vi "Shared Variables CD 2.0 Initialization VI.vi"(8 "error in (no error)":errorcluster, 10 "Custom XML":string, 11 "Device Item Ref in":T1 format="%.0x") -> (0 "error out":errorcluster, 3 "Device Item Ref out":T1 format="%.0x")   [LabVIEW 2017, in "Shared Variables CD 2.0 Configuration.lvlib"]
uses:
  Shared Variables CD 2.0 Configuration.lvlib
  <vilib>/NI Veristand/Custom Device API/Custom Device Item Ref.ctl
  <vilib>/NI Veristand/Custom Device API/Custom Device Channel.ctl
  <vilib>/NI Veristand/Custom Device API/Custom Device Channel Type.ctl
  Shared/Shared Variables CD 2.0 GUID Lookup.vi
  Shared/SV Global.vi
  <vilib>/NI VeriStand/Custom Device API/Custom Device API.lvlib
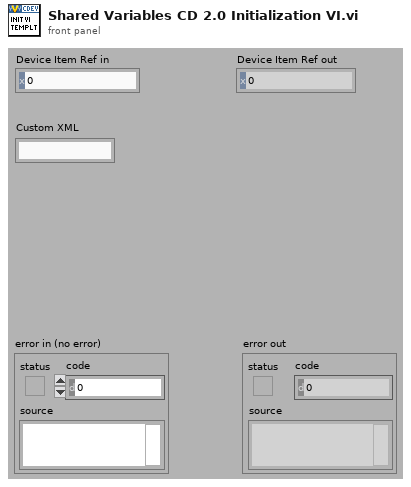
[diagram p1: front panel]
types:
  T1 = typedef "Custom Device API.lvlib/Custom Device Item Ref.ctl" = u64
  T2 = typedef "Custom Device API.lvlib/Custom Device Channel.ctl" = cluster{"Type":T3, "Units":string, "Default Value":dbl, "Faultable":bool, "Scalable":bool}
  T3 = typedef "Custom Device API.lvlib/Custom Device Channel Type.ctl" = enum16{"Input", "Output"}
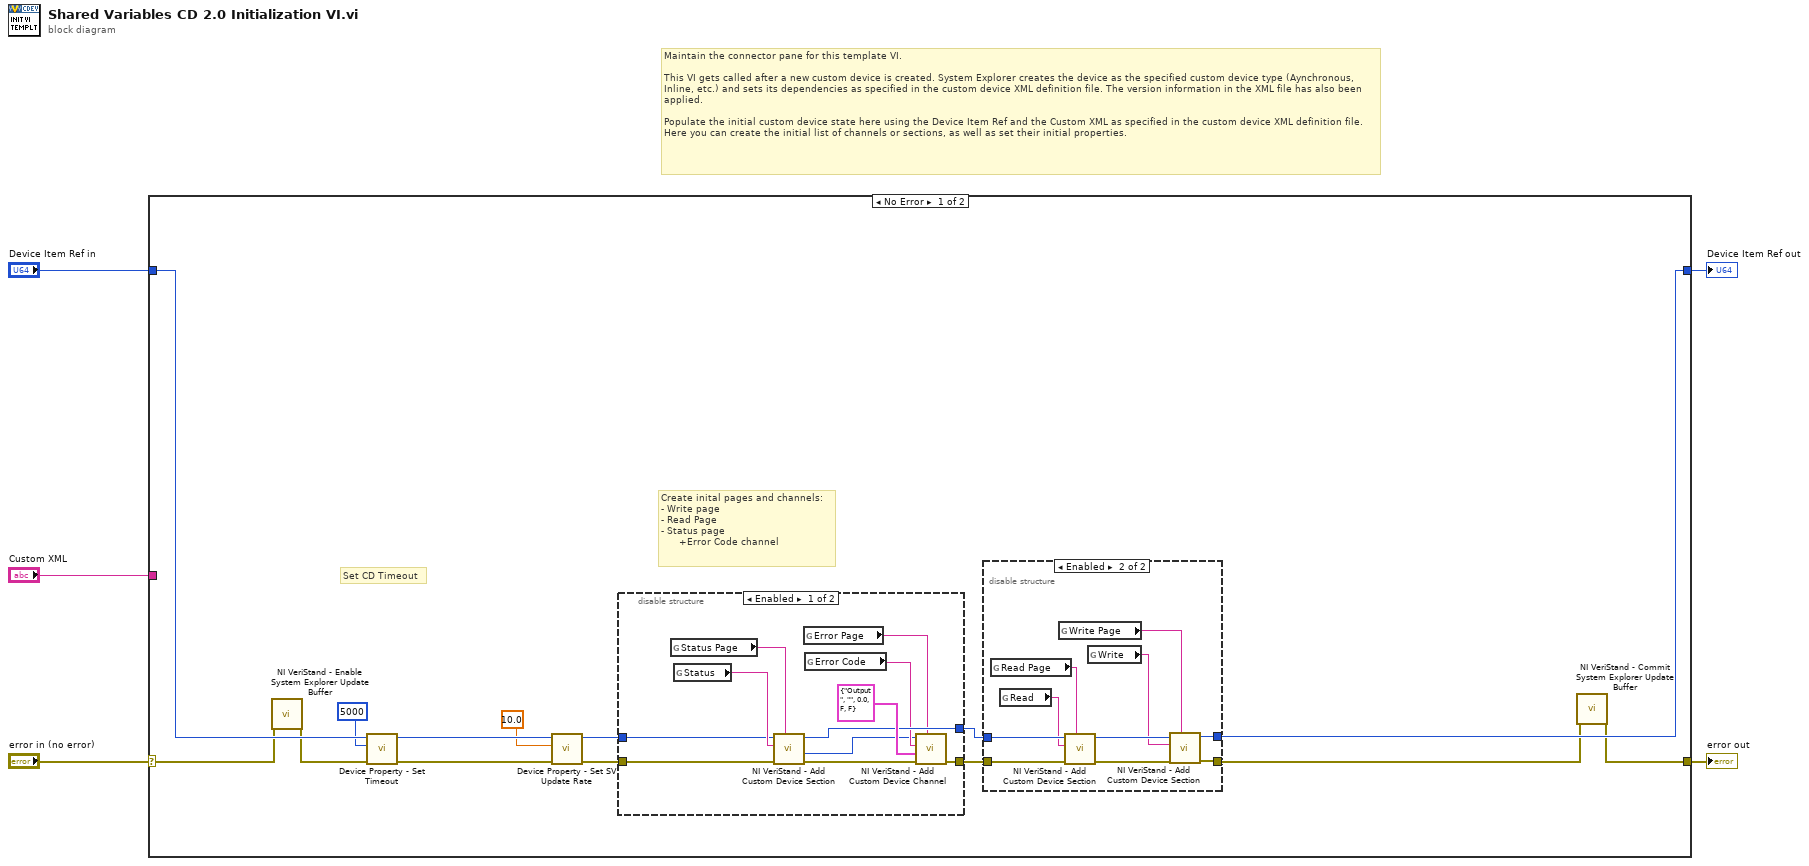
[diagram p0: block diagram]
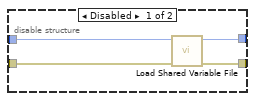
[diagram p3: hidden frame]
diagram:
  # "Maintain the connector pane for this template VI.\n\nThis VI gets called after a new custom device is created. System Explorer creates the device as the specified custom device type (Aynchronous, Inline, etc.) and sets its dependencies as specified in the custom device XML definition file. The version information in the XML file has also been applied.\n\nPopulate the initial custom device state here using the Device Item Ref and the Custom XML as specified in the custom device XML definition file. Here you can create the initial list of channels or sections, as well as set their initial properties."
  n1 = case shown="No Error" "error in (no error)" {
    selector: "error in (no error)" -> [w7 w48]
    tunnel: [w8 w48] -> w5
    tunnel: [w18 w47] -> w3
    tunnel: "Device Item Ref in" -> [w19 w47]
    tunnel: "Custom XML" -> [_ _]
    frame No Error {
      # "Set CD Timeout"
      # "Create inital pages and channels:\n- Write page\n- Read Page\n- Status page\n      +Error Code channel"
      n2 = call <vilib>:"NI VeriStand - Enable System Explorer Update Buffer.vi"("error in (no error)"=w7) -> ("error out"=w6:errorcluster)  [unwired: 10 in]
      n3 = call "Device Property - Set Timeout.vi"("error in (no error)"=w6, "Timout"=5000 ("IP Address"), "Device Ref in"=w19) -> ("error out"=w14:errorcluster, "Device Ref out"=w11:T1)  [unwired: 7 in]
      n4 = call "Device Property - Set SV Update Rate.vi"("error in (no error)"=w14, "Update Rate (ms)"=10.0 ("Value"), "Device Ref in"=w11) -> ("error out"=w13:errorcluster, "Item Ref out"=w12:T1)  [unwired: 7 in]
      n5 = disable-structure shown="Enabled" {
        disable-tunnel: [w29 w32] -> w16
        disable-tunnel: [w28 w31] -> w15
        disable-tunnel: w13 -> [w21 w31]
        disable-tunnel: w12 -> [w20 w32]
        frame Enabled {
          n6 = global read "Shared Variables CD 2.0 GUID Lookup.vi" "Status Page"() -> (w23:string)
          n7 = global read "SV Global.vi" "Status"() -> (w22:string)
          n8 = call <vilib>:"NI VeriStand - Add Custom Device Section.vi"("GUID (Default Section)"=w23, "error in (no error)"=w21, "Section Name"=w22, "Parent Ref in"=w20) -> ("error out"=w25:errorcluster, "Section Ptr"=w24:T1, "Parent Ref out"=w29:T1)  [unwired: 4 in, 1 out]
          n9 = global read "Shared Variables CD 2.0 GUID Lookup.vi" "Error Page"() -> (w27:string)
          n10 = global read "SV Global.vi" "Error Code"() -> (w26:string)
          n11 = call <vilib>:"NI VeriStand - Add Custom Device Channel.vi"("GUID (Default Channel)"=w27, "error in (no error)"=w25, "Channel"=T2 {"Type"=enum."Output", "Units"="", "Default Value"=0.0, "Faultable"=FALSE, "Scalable"=FALSE}, "Channel Name"=w26, "Parent Ref in"=w24) -> ("error out"=w28:errorcluster)  [unwired: 3 in, 3 out]
        }
        frame Disabled {
        }
      }
      n12 = disable-structure shown="Enabled" {
        disable-tunnel: [w36 w43] -> w18
        disable-tunnel: [w35 w41] -> w9
        disable-tunnel: w16 -> [w34 w46]
        disable-tunnel: w15 -> [w33 w45]
        frame Disabled {
          n13 = call "Load Shared Variable File.vi"("error in"=w33, "Device Ref in"=w34) -> ("error out"=w35:errorcluster, "Device Ref out"=w36:T1)  [unwired: 8 in]
        }
        frame Enabled {
          n14 = global read "Shared Variables CD 2.0 GUID Lookup.vi" "Read Page"() -> (w40:string)
          n15 = global read "SV Global.vi" "Read"() -> (w37:string)
          n16 = global read "Shared Variables CD 2.0 GUID Lookup.vi" "Write Page"() -> (w39:string)
          n17 = call <vilib>:"NI VeriStand - Add Custom Device Section.vi"("GUID (Default Section)"=w40, "error in (no error)"=w45, "Section Name"=w37, "Parent Ref in"=w46) -> ("error out"=w42:errorcluster, "Parent Ref out"=w44:T1)  [unwired: 4 in, 2 out]
          n18 = global read "SV Global.vi" "Write"() -> (w38:string)
          n19 = call <vilib>:"NI VeriStand - Add Custom Device Section.vi"("GUID (Default Section)"=w39, "error in (no error)"=w42, "Section Name"=w38, "Parent Ref in"=w44) -> ("error out"=w41:errorcluster, "Parent Ref out"=w43:T1)  [unwired: 4 in, 2 out]
        }
      }
      n20 = call <vilib>:"NI VeriStand - Commit System Explorer Update Buffer.vi"("error in (no error)"=w9) -> ("error out"=w8:errorcluster)  [unwired: 10 in]
    }
    frame Error {
    }
  }
  "error out" <- w5
  "Device Item Ref out" <- w3
